vi "Control 2-PID.vi"() -> ()   [LabVIEW 2011]
panel:
  out "Waveform Chart":sgl(graph)
  out "Error":dbl
  in  "Fuente Sur":refnum<visa-resource-name>="COM1"
  in  "Kd":dbl
  in  "Ki":dbl
  out "Tiempo de ejecución":dbl
  in  "stop":bool
  out "V":string
  in  "Kp":dbl
  in  "Temperatura deseada":dbl
  out "2":sgl(slide) min=0 max=100 scale=0.0..100.0 scale format="%.1f"
  out "1":sgl(slide) min=0 max=100 scale=0.0..200.0 scale format="%.1f"
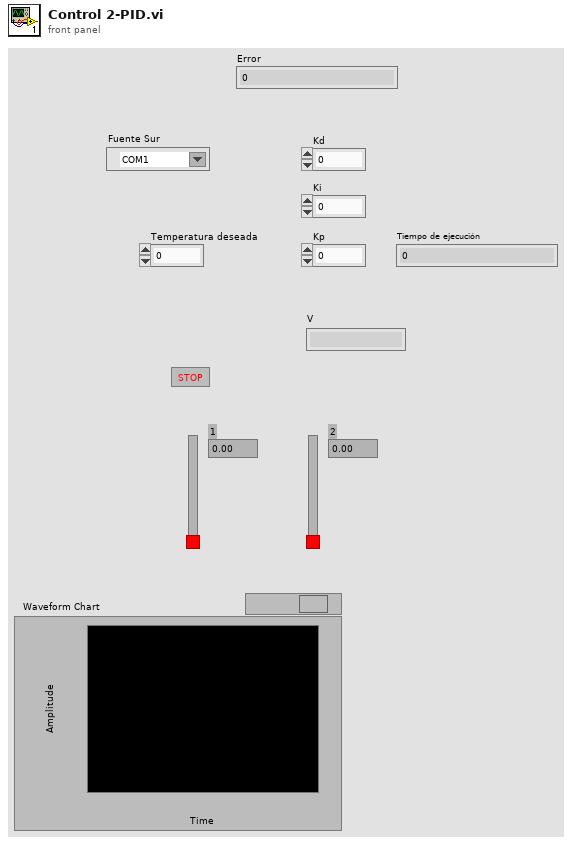
[diagram p1: front panel]
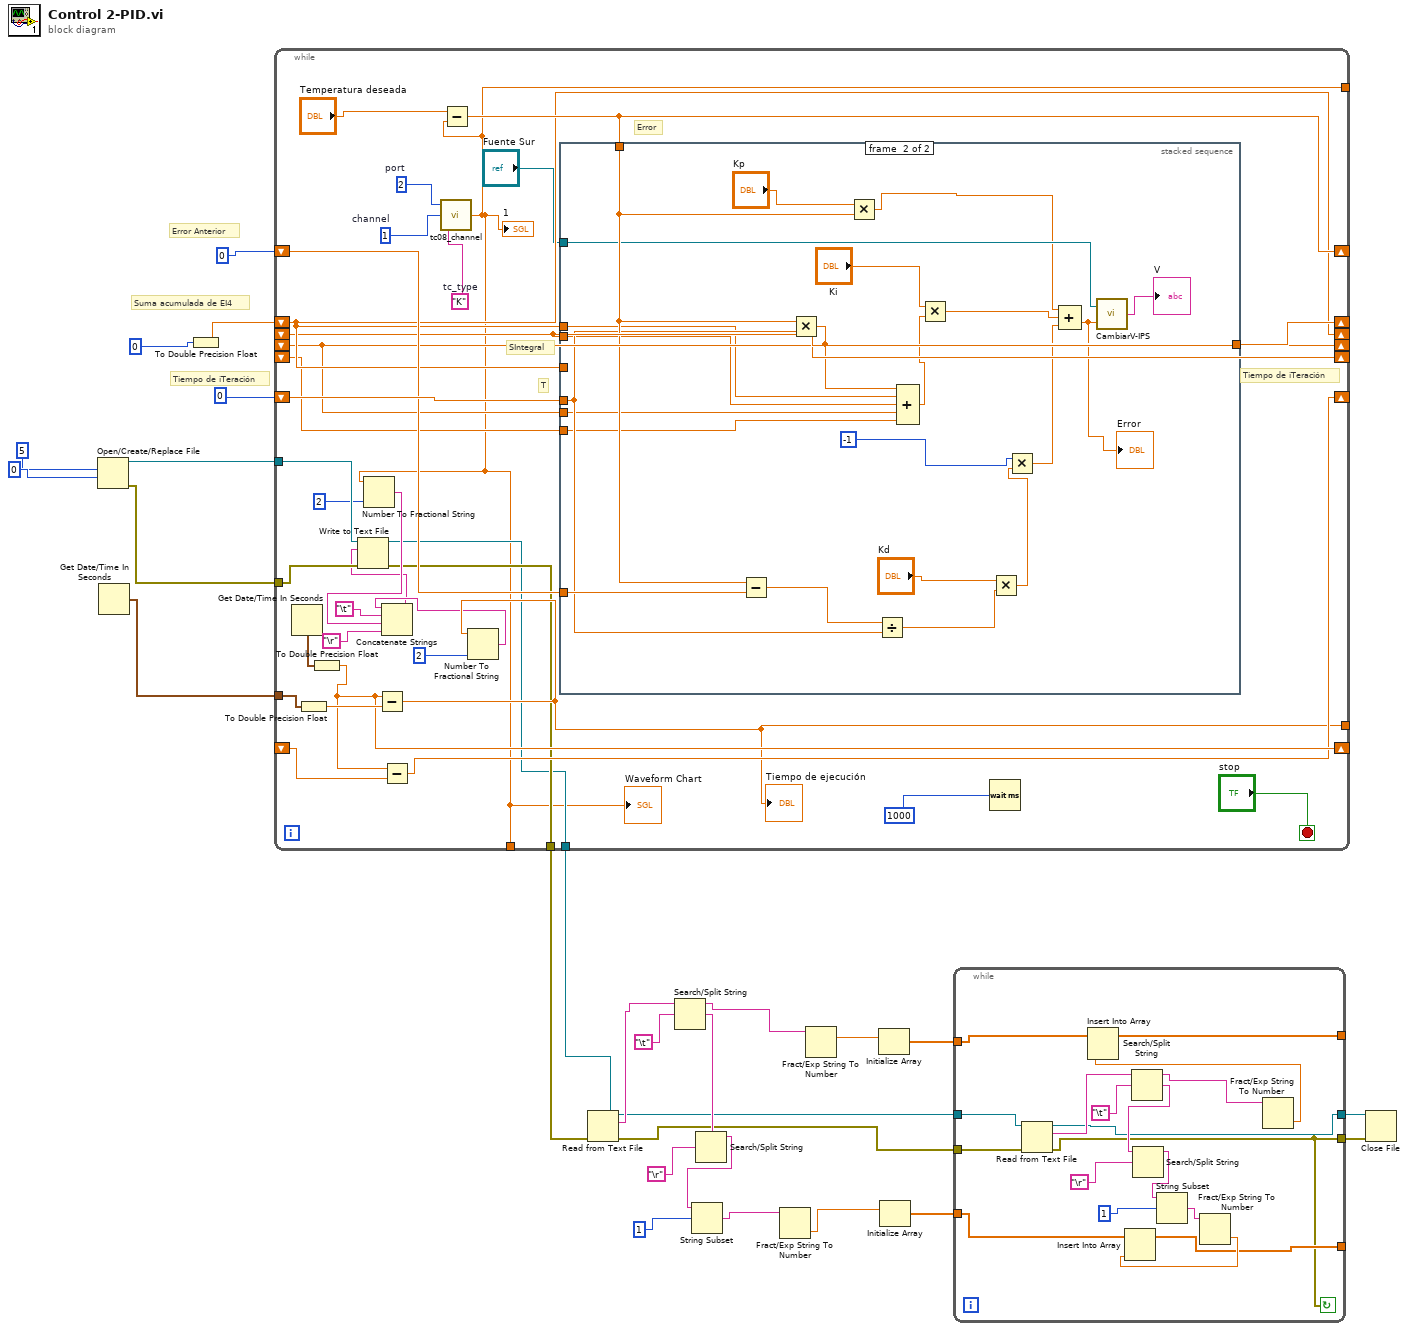
[diagram p0: block diagram]
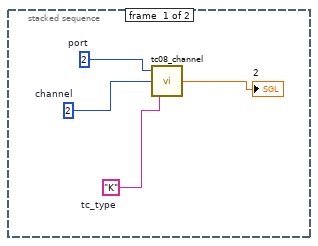
[diagram p2: hidden frame]
diagram:
  # "Suma acumulada de EI4"
  # "Error Anterior"
  # "Tiempo de iTeración"
  n1 = Open/Create/Replace File(operation (0:open)=5, access (0:read/write)=0) -> (refnum out=w19:refnum<file>, error out=w20:errorcluster)  [unwired: 4 in, 1 out]
  n2 = Get Date/Time In Seconds() -> (seconds since 1Jan1904=w27:timestamp)
  n3 = To Double Precision Float(number=0) -> (double precision float=w24:dbl)
  n4 = while {
    shift-right: [w47] -> _
    shift-left: w24 -> [w46]
    shift-right: [w50] -> _
    shift-left: 0 -> [w49]
    tunnel: w27 -> [w58]
    shift-right: [w56] -> _
    shift-left: _ -> [w57]
    shift-right: [w51] -> _
    shift-left: 0 -> [w48]
    shift-right: [w46] -> _
    shift-left: _ -> [w45]
    shift-right: [w45] -> _
    shift-left: _ -> [w44]
    shift-right: [w44] -> _
    shift-left: _ -> [w43]
    tunnel: [w40] -> _
    tunnel: [w28] -> _
    tunnel: w20 -> [w42]
    tunnel: w19 -> [w41]
    tunnel: [w35] -> w17
    tunnel: [w34] -> w18
    tunnel: [w28] -> _
    stop <- "stop" stop-if-true
    w52 = "K"  # tc_type
    w53 = u16 1  # channel
    w54 = u16 2  # port
    # "SIntegral"
    # "T"
    # "Error"
    # "Tiempo de iTeración"
    n5 = Get Date/Time In Seconds() -> (seconds since 1Jan1904=w60:timestamp)
    n6 = To Double Precision Float(number=w58) -> (double precision float=w59:dbl)
    n7 = To Double Precision Float(number=w60) -> (double precision float=w56:dbl)
    n8 = Subtract(x=w56, y=w59) -> (x-y=w40:dbl)
    "Tiempo de ejecución" <- w40
    n9 = Subtract(x=w56, y=w57) -> (x-y=w50:dbl)
    n10 = call "tc08_channel.vi"("tc_type"=w52, "channel"=w53, "port"=w54) -> ("Temperature"=w28:sgl)
    "1" <- w28
    "Waveform Chart" <- w28
    n11 = Number To Fractional String(number=w28, precision (6)=2) -> (F-format string=w37:string)  [unwired: 2 in]
    n12 = Subtract(x="Temperatura deseada", y=w28) -> (x-y=w51:dbl)
    n13 = Number To Fractional String(number=w40, precision (6)=2) -> (F-format string=w39:string)  [unwired: 2 in]
    n14 = Concatenate Strings(w39, "\t", w37, "\r") -> (w36:string)
    n15 = Write to Text File(file (use dialog)=w41, text=w36, error in=w42) -> (refnum out=w34:refnum<file>, error out=w35:errorcluster)  [unwired: 1 in, 1 out]
    n16 = stacked-sequence {
      tunnel: w51 -> [_ w80]
      tunnel: w46 -> [_ _]
      tunnel: w49 -> [_ w78]
      tunnel: w48 -> [_ w79]
      tunnel: [_ w76] -> w47
      tunnel: w46 -> [_ w75]
      tunnel: w45 -> [_ w74]
      tunnel: w44 -> [_ w73]
      tunnel: w43 -> [_ w72]
      tunnel: "Fuente Sur" -> [_ w71]
      frame #0 {
        w63 = "K"  # tc_type
        w64 = u16 2  # channel
        w65 = u16 2  # port
        n17 = call "tc08_channel.vi"("tc_type"=w63, "channel"=w64, "port"=w65) -> ("Temperature"=→"2":sgl)
      }
      frame #1 {
        n18 = Subtract(x=w80, y=w79) -> (x-y=w83:dbl)
        n19 = Multiply(x=w80, y=w78) -> (x*y=w76:dbl)
        n20 = Multiply(x="Kp", y=w80) -> (x*y=w69:dbl)
        n21 = Divide(x=w83, y=w78) -> (x/y=w84:dbl)
        n22 = Compound Arithmetic op=ADD(w76, w75, w74, w73, w72) -> (w77:dbl)
        n23 = Multiply(x="Ki", y=w77) -> (x*y=w82:dbl)
        n24 = Multiply(x="Kd", y=w84) -> (x*y=w68:dbl)
        n25 = Multiply(x=-1, y=w68) -> (x*y=w67:dbl)
        n26 = Compound Arithmetic op=ADD(w69, w82, w67) -> (w70:dbl)
        "Error" <- w70
        n27 = call "CambiarV-IPS.vi"("Numeric"=w70, "VISA resource name"=w71) -> ("Voltios"=→"V":string)
      }
    }
    n28 = Wait (ms)(milliseconds to wait=1000) -> ()  [unwired: 1 out]
  }
  n29 = Read from Text File(file (use dialog)=w18, error in=w17) -> (refnum out=w6:refnum<file>, text=w12:string, error out=w5:errorcluster)  [unwired: 2 in, 1 out]
  n30 = Search/Split String(string=w12, search string/char (-)="\t") -> (substring before match=w13:string, match + rest of string=w10:string)  [unwired: 1 in, 1 out]
  n31 = Search/Split String(string=w10, search string/char (-)="\r") -> (substring before match=w8:string)  [unwired: 1 in, 2 out]
  n32 = String Subset(string=w8, offset (0)=1) -> (substring=w15:string)  [unwired: 1 in]
  n33 = Fract/Exp String To Number(string=w15) -> (number=w14:dbl)  [unwired: 3 in, 1 out]
  n34 = Fract/Exp String To Number(string=w13) -> (number=w16:dbl)  [unwired: 3 in, 1 out]
  n35 = Initialize Array(w16) -> (w4:dbl[])  [unwired: 1 in]
  n36 = Initialize Array(w14) -> (w3:dbl[])  [unwired: 1 in]
  n37 = while {
    tunnel: w6 -> [w105]
    tunnel: w5 -> [w104]
    tunnel: w4 -> [w103]
    tunnel: w3 -> [w102]
    tunnel: [w91] -> _
    tunnel: [w90] -> _
    tunnel: [w88] -> w2
    tunnel: [w89] -> w1
    stop <- w88 continue-if-true
    n38 = Read from Text File(file (use dialog)=w105, error in=w104) -> (refnum out=w89:refnum<file>, text=w99:string, error out=w88:errorcluster)  [unwired: 2 in, 1 out]
    n39 = Search/Split String(string=w99, search string/char (-)="\t") -> (substring before match=w101:string, match + rest of string=w98:string)  [unwired: 1 in, 1 out]
    n40 = Search/Split String(string=w98, search string/char (-)="\r") -> (substring before match=w95:string)  [unwired: 1 in, 2 out]
    n41 = String Subset(string=w95, offset (0)=1) -> (substring=w93:string)  [unwired: 1 in]
    n42 = Fract/Exp String To Number(string=w93) -> (number=w92:dbl)  [unwired: 3 in, 1 out]
    n43 = Insert Into Array(array=w102, new element=w92) -> (w91:dbl[])  [unwired: 1 in]
    n44 = Fract/Exp String To Number(string=w101) -> (number=w94:dbl)  [unwired: 3 in, 1 out]
    n45 = Insert Into Array(array=w103, new element=w94) -> (w90:dbl[])  [unwired: 1 in]
  }
  n46 = Close File(refnum=w1, error in=w2) -> ()  [unwired: 2 out]
